vi "Conditioning.vi"() -> ()   [LabVIEW 2014]
uses:
  Licker.lvclass
  Juicer.lvclass
  Acquisition.lvclass
  Stimulus.lvclass
panel:
  out "Number of Licks":dbl[](array[numeric]) caption="#Licks"
  in  "LICK":bool[](array[boolean])=[FALSE, FALSE, FALSE, FALSE, FALSE]
  out "Last lick":timestamp[](array[timestamp])
  in  "IRI":dbl[](array[numeric]) caption="IRI (msec)"
  out "Time to stimulation":dbl[](array[numeric]) caption="Time to Stim"
  out "Rewards Given":dbl[](array[numeric]) caption="#Rew"
  in  "microL_per_pulse":dbl[](array[numeric]) caption="ml/p"
  in  "Pulse Duration":dbl[](array[numeric]) caption="Pulse (ms)"
  in  "Thr":dbl[](array[numeric])=[10.0, 10.0, 10.0, 10.0, 10.0]
  out "Water":bool[](array[boolean])
  out "Licks":bool[](array[boolean])
  out "error out":errorcluster
  in  "ITI":dbl[](array[numeric]) caption="ITI (min)"
  out "Stimulus":i32
  in  "RUN":bool[](array[boolean])=[FALSE, FALSE, FALSE, FALSE, FALSE]
  out "Licker":i32
  out "Acquisition":i32
  out "Juicer":i32
  in  "REC":bool[](array[boolean])=[FALSE, FALSE, FALSE, FALSE, FALSE]
  in  "liquid_type":string(combo)="water"
  in  "Type":enum16{"Calibrate", "Freerun", "BW"}[](array[ring])
  out "Optical traces":waveform(dbl)[](graph)
  in  "Mice ID":dbl[](array[numeric])
  in  "Stop":bool
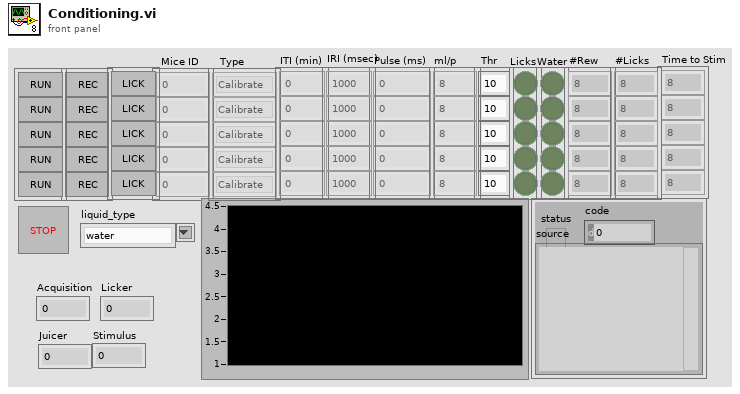
[diagram p1: front panel]
types:
  T1 = enum16{"stim_periods", "licks", "liquid_delivery"}
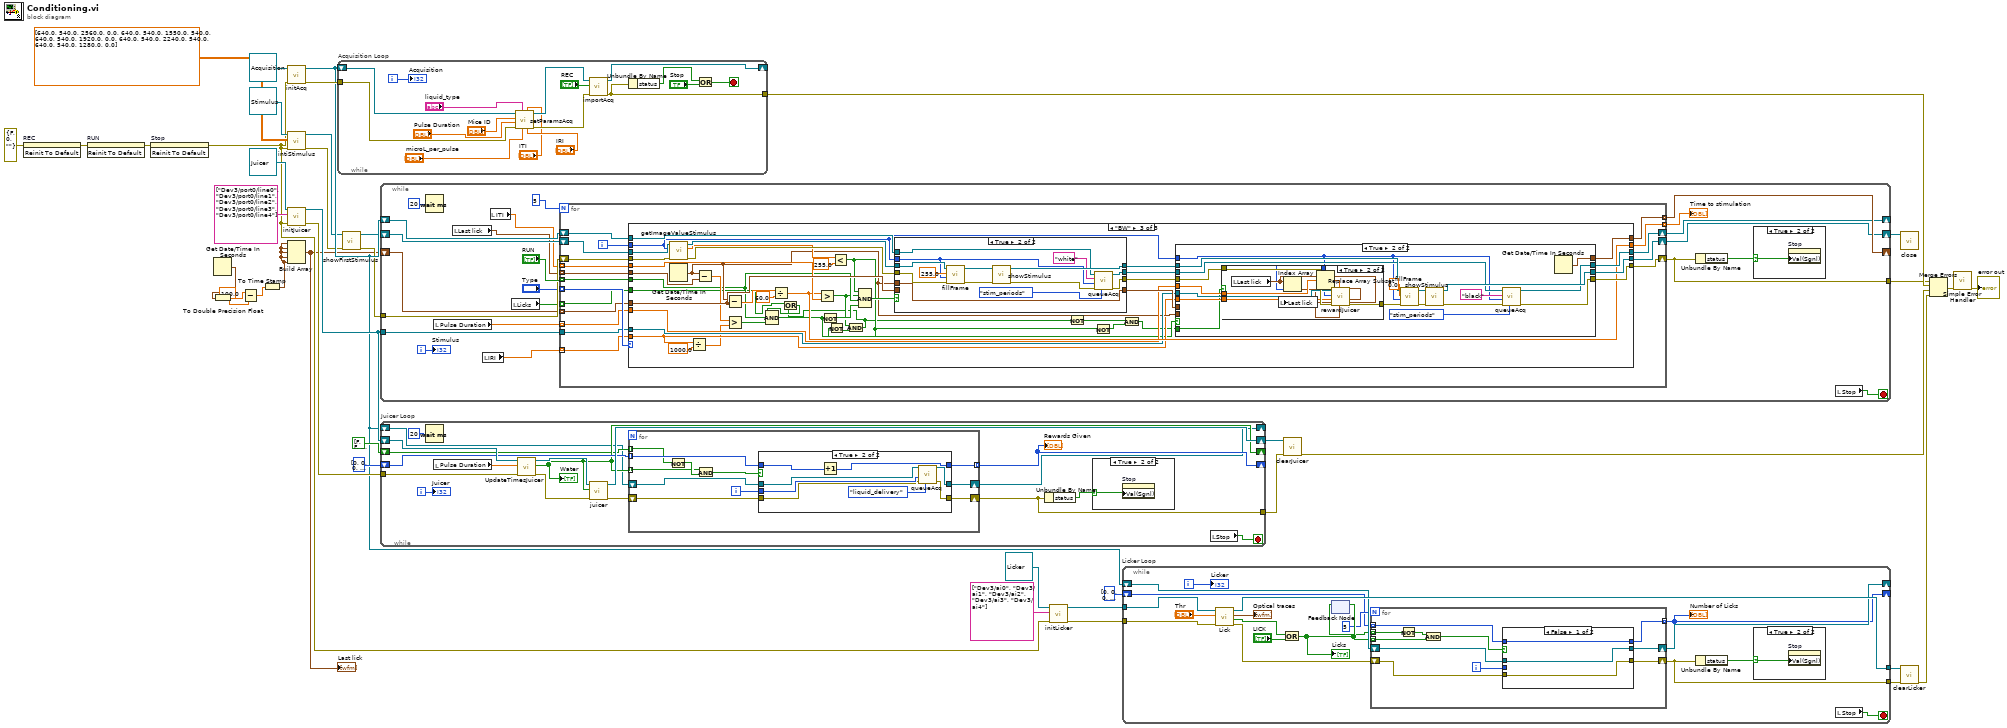
[diagram p0: block diagram]
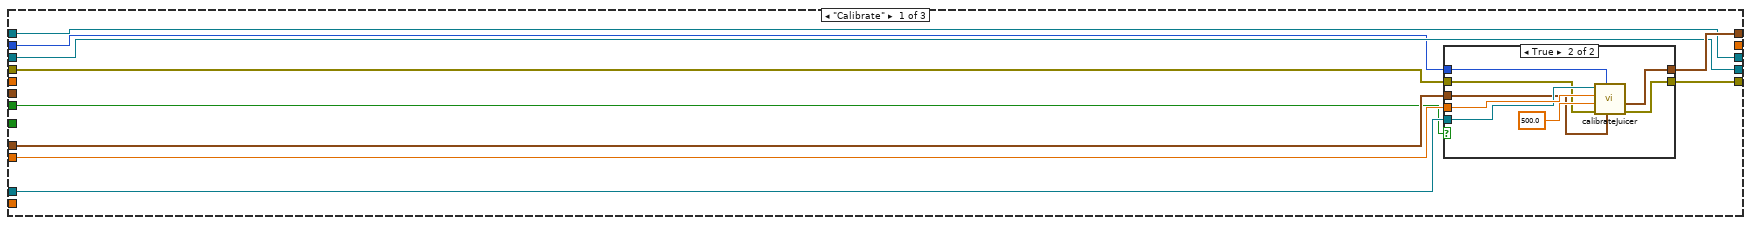
[diagram p3: hidden frame]
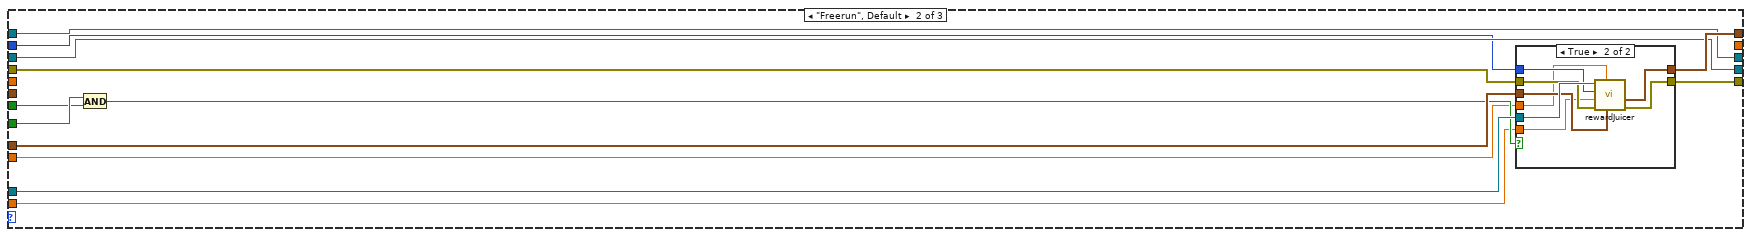
[diagram p5: hidden frame]
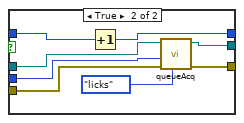
[diagram p11: hidden frame]
diagram:
  n1 = invoke on="REC" class="Arr (strict)" method="Reinit To Default"(error in=errorcluster {"status"=FALSE, "code"=0, "source"=""} ("error in (no error)")) -> (error out=w15:errorcluster)  [unwired: 2 in, 2 out]
  n2 = invoke on="RUN" class="Arr (strict)" method="Reinit To Default"(error in=w15) -> (error out=w14:errorcluster)  [unwired: 2 in, 2 out]
  n3 = invoke on="Stop" class="Bool (strict)" method="Reinit To Default"(error in=w14) -> (error out=w12:errorcluster)  [unwired: 2 in, 2 out]
  n4 = Get Date/Time In Seconds() -> (seconds since 1Jan1904=w4:timestamp)
  n5 = To Double Precision Float(number=w4) -> (double precision float=w3:dbl)
  n6 = Subtract(x=w3, y=100.0) -> (x-y=w1:dbl)
  n7 = To Time Stamp(1:w1) -> (0:w5:timestamp)
  n8 = call-dynamic "initAcq.vi"("error in (no error)"=w12, "Acquisition in"=refnum<class "Acquisition.lvclass"> refnum ("Acquisition.lvclass")) -> ("error out"=w32:errorcluster, "Acquisition out"=w16:refnum<class "Acquisition.lvclass">)  [unwired: 8 in]
  n9 = call-dynamic "intiStimulus.vi"("error in (no error)"=w12, "Monitor parameters"=dbl[][] [[640.0, 540.0, 2560.0, 0.0], [640.0, 540.0, 1550.0, 540.0], [640.0, 540.0, 1920.0, 0.0], [640.0, 540.0, 2240.0, 540.0], [640.0, 540.0, 1280.0, 0.0]], "Stimulus in"=refnum<class "Stimulus.lvclass"> refnum ("Stimulus.lvclass")) -> ("error out"=w10:errorcluster, "Stimulus out"=w11:refnum<class "Stimulus.lvclass">)  [unwired: 7 in]
  n10 = call-dynamic "initJuicer.vi"("error in (no error)"=w12, "Lines"=string[] ["Dev3/port0/line0", "Dev3/port0/line1", "Dev3/port0/line2", "Dev3/port0/line3", "Dev3/port0/line4"], "Juicer in"=refnum<class "Juicer.lvclass"> refnum ("Juicer.lvclass")) -> ("error out"=w36:errorcluster, "Juicer out"=w22:refnum<class "Juicer.lvclass">)  [unwired: 7 in]
  n11 = Build Array(w5, w5, w5, w5, w5) -> (w7:timestamp[])
  "Last lick" <- w7
  n12 = while "Acquisition Loop" {
    tunnel: w32 -> [w51]
    tunnel: [w45] -> w28
    shift-right: [w46] -> _
    shift-left: w16 -> [w58]
    i -> [w47]
    stop <- w49 stop-if-true
    n13 = call-dynamic "setParamsAcq.vi"("IRI"="IRI", "ITI"="ITI", "microL_per_pulse"="microL_per_pulse", "liquid_type"="liquid_type", "error in (no error)"=w51, "Pulse Duration"="Pulse Duration", "Mice ID"="Mice ID", "Acquisition in"=w58) -> ("error out"=w52:errorcluster, "Acquisition out"=w57:refnum<class "Acquisition.lvclass">)  [unwired: 2 in]
    n14 = call-dynamic "importAcq.vi"("error in (no error)"=w52, "REC"="REC", "Acquisition in"=w57) -> ("error out"=w45:errorcluster, "Acquisition out"=w46:refnum<class "Acquisition.lvclass">)  [unwired: 7 in]
    n15 = Unbundle By Name(w45) -> ("status"=w44:bool)
    n16 = Or(x=w44, y="Stop") -> (x .or. y?=w49:bool)
    "Acquisition" <- w47
  }
  n17 = call-dynamic "showFirstStimulus.vi"("error in (no error)"=w10, "Stimulus in"=w11) -> ("error out"=w9:errorcluster, "Stimulus out"=w8:refnum<class "Stimulus.lvclass">)  [unwired: 8 in]
  n18 = while {
    tunnel: w22 -> [w79]
    tunnel: w9 -> [w78]
    shift-right: [w74] -> _
    shift-left: w7 -> [w75]
    tunnel: [w62] -> w18
    shift-right: [w66] -> _
    shift-left: w16 -> [w67]
    shift-right: [w71] -> w19
    shift-left: w8 -> [w72]
    i -> [w69]
    stop <- w70 stop-if-true
    n19 = Wait (ms)(milliseconds to wait=u32 20) -> ()  [unwired: 1 out]
    n20 = local read "Pulse Duration"() -> (w77:dbl[])
    n21 = local read "Last lick"() -> (w64:timestamp[])
    n22 = local read "IRI"() -> (w60:dbl[])
    n23 = local read "ITI"() -> (w59:dbl[])
    n24 = local read "Licks"() -> (w76:bool[])
    n25 = for {
      N: 5 -> [_]
      tunnel: "RUN" -> [w92] mode=indexing
      tunnel: "Type" -> [w99] mode=indexing
      tunnel: w79 -> [w98]
      tunnel: w77 -> [w96] mode=indexing
      tunnel: w76 -> [w95] mode=indexing
      tunnel: w75 -> [w94] mode=indexing
      tunnel: [w93] -> w74 mode=indexing
      shift-right: [w89] -> w62
      shift-left: w78 -> [w97]
      tunnel: w59 -> [w87] mode=indexing
      shift-right: [w86] -> w66
      shift-left: w67 -> [w85]
      shift-right: [w90] -> w71
      shift-left: w72 -> [w91]
      tunnel: [w84] -> w65 mode=indexing
      tunnel: w60 -> [w83] mode=indexing
      tunnel: w64 -> [w82] mode=indexing
      i -> [w88]
      n26 = case shown="\"BW\"" w99 {
        tunnel: [w106 w130 w181] -> w89
        tunnel: w97 -> [w107 w131 w167]
        tunnel: w98 -> [w108 w132 w171]
        tunnel: w96 -> [w109 w120 w170]
        tunnel: w95 -> [_ w126 w151]
        tunnel: w94 -> [w105 w129 w182]
        tunnel: [w104 w128 w180] -> w93
        tunnel: w92 -> [w103 w125 w157]
        tunnel: w91 -> [w102 w124 w169]
        tunnel: [w102 w124 w179] -> w90
        tunnel: w88 -> [w100 w123 w162]
        tunnel: w85 -> [w101 w122 w178]
        tunnel: w87 -> [_ _ w176]
        tunnel: [w101 w122 w175] -> w86
        tunnel: [_ _ w172] -> w84
        tunnel: w83 -> [_ w121 w154]
        tunnel: w82 -> [_ _ w159]
        frame "Calibrate" {
          n27 = case shown="True" w103 {
            tunnel: w109 -> [_ w119]
            tunnel: w108 -> [_ w117]
            tunnel: w107 -> [w110 w116]
            tunnel: [w110 w115] -> w106
            tunnel: w105 -> [w111 w114]
            tunnel: [w111 w113] -> w104
            tunnel: w100 -> [_ w112]
            frame False {
            }
            frame True {
              n28 = call-dynamic "calibrateJuicer.vi"("Time Stamp"=w114, "Window Number (0...15)"=w112, "error in (no error)"=w116, "ISI"=500.0, "Pulse duration"=w119, "Juicer in"=w117) -> ("error out"=w115:errorcluster, "Time Stamp 2"=w113:timestamp)  [unwired: 3 in, 1 out]
            }
          }
        }
        frame "Freerun", Default {
          n29 = And(x=w126, y=w125) -> (x .and. y?=w127:bool)
          n30 = case shown="True" w127 {
            tunnel: w132 -> [_ w142]
            tunnel: w123 -> [_ w141]
            tunnel: w131 -> [w134 w140]
            tunnel: [w134 w139] -> w130
            tunnel: w129 -> [w133 w138]
            tunnel: [w133 w137] -> w128
            tunnel: w121 -> [_ w136]
            tunnel: w120 -> [_ w135]
            frame False {
            }
            frame True {
              n31 = call-dynamic "rewardJuicer.vi"("seconds since 1Jan1904 2"=w138, "pulse dur"=w135, "error in (no error)"=w140, "IRI"=w136, "Window Number (0...15)"=w141, "Juicer in"=w142) -> ("error out"=w139:errorcluster, "seconds since 1Jan1904"=w137:timestamp)  [unwired: 3 in, 1 out]
            }
          }
        }
        frame "BW" {
          n32 = call-dynamic "getImageValueStimulus.vi"("error in (no error)"=w167, "index"=w162, "Stimulus in"=w169) -> ("error out"=w166:errorcluster, "Pixel Value (Float)"=w164:sgl, "Stimulus out"=w168:refnum<class "Stimulus.lvclass">)  [unwired: 6 in]
          n33 = Get Date/Time In Seconds() -> (seconds since 1Jan1904=w161:timestamp)
          n34 = Divide(x=w154, y=1000.0) -> (x/y=w153:dbl)
          n35 = Subtract(x=w161, y=w159) -> (x-y=w160:dbl)
          n36 = Subtract(x=w161, y=w182) -> (x-y=w174:dbl)
          n37 = Greater?(x=w160, y=w153) -> (0:w158:bool)
          n38 = Divide(x=w174, y=60.0) -> (x/y=w172:dbl)
          n39 = Greater?(x=w172, y=w176) -> (0:w149:bool)
          n40 = Less?(x=w164, y=sgl 255.0) -> (x < y?=w147:bool)
          n41 = Not(x=w147) -> (.not. x?=w148:bool)
          n42 = And(x=w149, y=w148) -> (x .and. y?=w144:bool)
          n43 = Or(x=w151, y=w144) -> (x .or. y?=w150:bool)
          n44 = Compound Arithmetic op=AND(w150, w157, w158) -> (w152:bool)
          n45 = Not(x=w152) -> (.not. x?=w156:bool)
          n46 = Compound Arithmetic op=AND(w147, w149, w157, w156) -> (w165:bool)
          n47 = case shown="True" w165 {
            tunnel: [w221 w237] -> w185
            tunnel: [w222 w228] -> w184
            tunnel: w182 -> [w223 _]
            tunnel: [w223 w233] -> w183
            tunnel: w161 -> [_ w233]
            tunnel: w166 -> [w222 w232]
            tunnel: w168 -> [w221 w231]
            tunnel: w162 -> [_ w230]
            tunnel: w178 -> [w220 w227]
            tunnel: [w220 w226] -> w177
            frame False {
            }
            frame True {
              n48 = call-dynamic "fillFrame.vi"("error in (no error)"=w232, "index"=w230, "Pixel Value (U8, U16, I16, Float)"=sgl 255.0, "Stimulus in"=w231) -> ("error out"=w234:errorcluster, "Stimulus out"=w236:refnum<class "Stimulus.lvclass">)  [unwired: 6 in]
              n49 = call-dynamic "showStimulus.vi"("error in (no error)"=w234, "Stimulus in"=w236) -> ("error out"=w229:errorcluster, "Stimulus out"=w237:refnum<class "Stimulus.lvclass">)  [unwired: 8 in]
              n50 = call-dynamic "queueAcq.vi"("table"=T1."stim_periods", "error in (no error)"=w229, "Window Number (0...15)"=w230, "period_type"="white", "Acquisition in"=w227) -> ("error out"=w228:errorcluster, "Acquisition out"=w226:refnum<class "Acquisition.lvclass">)  [unwired: 4 in, 1 out]
            }
          }
          n51 = Not(x=w144) -> (.not. x?=w143:bool)
          n52 = Not(x=w147) -> (.not. x?=w146:bool)
          n53 = And(x=w143, y=w146) -> (x .and. y?=w145:bool)
          n54 = case shown="True" w152 {
            tunnel: w185 -> [w189 w205]
            tunnel: [w189 w204] -> w179
            tunnel: w184 -> [w188 w196]
            tunnel: [w188 w201] -> w181
            tunnel: [w187 w203] -> w180
            tunnel: w183 -> [w187 _]
            tunnel: w177 -> [w186 w200]
            tunnel: w162 -> [_ w191]
            tunnel: [w186 w197] -> w175
            tunnel: w171 -> [_ w194]
            tunnel: w161 -> [_ _]
            tunnel: w170 -> [_ w193]
            tunnel: w154 -> [_ w192]
            tunnel: w145 -> [_ w190]
            frame False {
            }
            frame True {
              n55 = case shown="True" w190 {
                tunnel: w196 -> [w209 w219]
                tunnel: [w209 w218] -> w195
                tunnel: w194 -> [_ w217]
                tunnel: w193 -> [_ w216]
                tunnel: w192 -> [_ w215]
                tunnel: w191 -> [_ w211]
                frame False {
                }
                frame True {
                  n56 = local read "Last lick"() -> (w212:timestamp[])
                  n57 = Index Array(array=w212, index=w211) -> (element=w210:timestamp)
                  n58 = call-dynamic "rewardJuicer.vi"("seconds since 1Jan1904 2"=w210, "pulse dur"=w216, "error in (no error)"=w219, "IRI"=w215, "Window Number (0...15)"=w211, "Juicer in"=w217) -> ("error out"=w218:errorcluster, "seconds since 1Jan1904"=w213:timestamp)  [unwired: 3 in, 1 out]
                  n59 = Replace Array Subset(array=w212, new element=w213, index=w211) -> (w214:timestamp[])
                  n60 = local write "Last lick"(w214) -> ()
                }
              }
              n61 = call-dynamic "fillFrame.vi"("error in (no error)"=w195, "index"=w191, "Pixel Value (U8, U16, I16, Float)"=sgl 0.0, "Stimulus in"=w205) -> ("error out"=w206:errorcluster, "Stimulus out"=w208:refnum<class "Stimulus.lvclass">)  [unwired: 6 in]
              n62 = call-dynamic "showStimulus.vi"("error in (no error)"=w206, "Stimulus in"=w208) -> ("error out"=w202:errorcluster, "Stimulus out"=w204:refnum<class "Stimulus.lvclass">)  [unwired: 8 in]
              n63 = call-dynamic "queueAcq.vi"("table"=T1."stim_periods", "error in (no error)"=w202, "Window Number (0...15)"=w191, "period_type"="black", "Acquisition in"=w200) -> ("error out"=w201:errorcluster, "Acquisition out"=w197:refnum<class "Acquisition.lvclass">)  [unwired: 4 in, 1 out]
              n64 = Get Date/Time In Seconds() -> (seconds since 1Jan1904=w203:timestamp)
            }
          }
        }
      }
    }
    "Time to stimulation" <- w65
    n65 = Unbundle By Name(w62) -> ("status"=w61:bool)
    n66 = case shown="True" w61 {
      selector: w61 -> [_ w81]
      frame False {
      }
      frame True {
        n67 = property on="Stop" class="Bool (strict)"("Val(Sgnl)"=w81) -> ()  [unwired: 2 in, 2 out]
      }
    }
    n68 = local read "Stop"() -> (w70:bool)
    "Stimulus" <- w69
  }
  n69 = while "Juicer Loop" {
    tunnel: [w245] -> w37
    tunnel: w36 -> [w250]
    shift-right: [w252] -> w38
    shift-left: w22 -> [w253]
    shift-right: [w242] -> _
    shift-left: i32[] [0, 0, 0, 0, 0] ("Array") -> [w243]
    shift-right: [w241] -> _
    shift-left: bool[] [FALSE, FALSE, FALSE, FALSE, FALSE] ("Juice") -> [w240]
    shift-right: [w238] -> _
    shift-left: w16 -> [w239]
    i -> [w246]
    stop <- w255 stop-if-true
    n70 = Wait (ms)(milliseconds to wait=u32 20) -> ()  [unwired: 1 out]
    n71 = local read "Pulse Duration"() -> (w247:dbl[])
    n72 = call-dynamic "UpdateTimesJuicer.vi"("error in (no error)"=w250, "Pulse Duration"=w247, "Juicer in"=w253) -> ("error out"=w251:errorcluster, "Juice"=w241:bool[], "Juicer out"=w254:refnum<class "Juicer.lvclass">)  [unwired: 6 in]
    "Water" <- w241
    n73 = call-dynamic "juicer.vi"("error in (no error)"=w251, "data"=w241, "Juicer in"=w254) -> ("error out"=w249:errorcluster, "Juicer out"=w252:refnum<class "Juicer.lvclass">)  [unwired: 7 in]
    n74 = for {
      tunnel: w241 -> [w265] mode=indexing
      shift-right: [w263] -> w245
      shift-left: w249 -> [w264]
      tunnel: w243 -> [w262] mode=indexing
      tunnel: [w261] -> w242 mode=indexing
      tunnel: w240 -> [w260] mode=indexing
      shift-right: [w258] -> w238
      shift-left: w239 -> [w259]
      i -> [w257]
      n75 = Not(x=w260) -> (.not. x?=w266:bool)
      n76 = And(x=w265, y=w266) -> (x .and. y?=w267:bool)
      n77 = case shown="True" w267 {
        tunnel: w257 -> [_ w277]
        tunnel: w264 -> [w270 w276]
        tunnel: [w270 w275] -> w263
        tunnel: w262 -> [w269 w274]
        tunnel: [w269 w273] -> w261
        tunnel: w259 -> [w268 w272]
        tunnel: [w268 w271] -> w258
        frame False {
        }
        frame True {
          n78 = Increment(x=w274) -> (x+1=w273:i32)
          n79 = call-dynamic "queueAcq.vi"("table"=T1."liquid_delivery", "error in (no error)"=w276, "Window Number (0...15)"=w277, "Acquisition in"=w272) -> ("error out"=w275:errorcluster, "Acquisition out"=w271:refnum<class "Acquisition.lvclass">)  [unwired: 5 in, 1 out]
        }
      }
    }
    "Rewards Given" <- w242
    n80 = Unbundle By Name(w245) -> ("status"=w244:bool)
    n81 = case shown="True" w244 {
      selector: w244 -> [_ w256]
      frame False {
      }
      frame True {
        n82 = property on="Stop" class="Bool (strict)"("Val(Sgnl)"=w256) -> ()  [unwired: 2 in, 2 out]
      }
    }
    n83 = local read "Stop"() -> (w255:bool)
    "Juicer" <- w246
  }
  n84 = call-dynamic "initLicker.vi"("error in (no error)"=w12, "Lines"=string[] ["Dev3/ai0", "Dev3/ai1", "Dev3/ai2", "Dev3/ai3", "Dev3/ai4"], "Licker in"=refnum<class "Licker.lvclass"> refnum ("Licker.lvclass")) -> ("error out"=w34:errorcluster, "Licker out"=w39:refnum<class "Licker.lvclass">)  [unwired: 7 in]
  n85 = while "Licker Loop" {
    tunnel: w34 -> [w294]
    tunnel: [w279] -> w31
    tunnel: w39 -> [w296]
    tunnel: [w295] -> w35
    shift-right: [w286] -> _
    shift-left: w16 -> [w287]
    shift-right: [w280] -> _
    shift-left: i32[] [0, 0, 0, 0, 0] ("Array") -> [w281]
    i -> [w290]
    stop <- w297 stop-if-true
    n86 = call-dynamic "Lick.vi"("error in (no error)"=w294, "% decrease Thr"="Thr", "Licker in"=w296) -> ("error out"=w291:errorcluster, "Lick?"=w288:bool[], "data"=→"Optical traces":waveform(dbl)[], "Licker out"=w295:refnum<class "Licker.lvclass">)  [unwired: 5 in]
    n87 = Or(x=w288, y="LICK") -> (x .or. y?=w285:bool[])
    "Licks" <- w285
    n88 = feedback-in #1(w285) -> ()
    n89 = feedback #1() -> (w284:bool[])  [unwired: 1 in]
    n90 = for {
      N: 5 -> [_]
      tunnel: w285 -> [w304] mode=indexing
      shift-right: [w308] -> w279
      shift-left: w291 -> [w309]
      shift-right: [w306] -> w286
      shift-left: w287 -> [w307]
      tunnel: w284 -> [w303] mode=indexing
      tunnel: w281 -> [w300] mode=indexing
      tunnel: [w299] -> w280 mode=indexing
      i -> [w305]
      n91 = Not(x=w303) -> (.not. x?=w302:bool)
      n92 = And(x=w302, y=w304) -> (x .and. y?=w301:bool)
      n93 = case shown="False" w301 {
        tunnel: w305 -> [_ w315]
        tunnel: w309 -> [w312 w319]
        tunnel: [w312 w318] -> w308
        tunnel: w307 -> [w311 w317]
        tunnel: [w311 w316] -> w306
        tunnel: w300 -> [w310 w314]
        tunnel: [w310 w313] -> w299
        frame False {
        }
        frame True {
          n94 = Increment(x=w314) -> (x+1=w313:i32)
          n95 = call-dynamic "queueAcq.vi"("table"=T1."licks", "error in (no error)"=w319, "Window Number (0...15)"=w315, "Acquisition in"=w317) -> ("error out"=w318:errorcluster, "Acquisition out"=w316:refnum<class "Acquisition.lvclass">)  [unwired: 5 in, 1 out]
        }
      }
    }
    "Number of Licks" <- w280
    n96 = Unbundle By Name(w279) -> ("status"=w289:bool)
    n97 = case shown="True" w289 {
      selector: w289 -> [_ w298]
      frame False {
      }
      frame True {
        n98 = property on="Stop" class="Bool (strict)"("Val(Sgnl)"=w298) -> ()  [unwired: 2 in, 2 out]
      }
    }
    n99 = local read "Stop"() -> (w297:bool)
    "Licker" <- w290
  }
  n100 = call-dynamic "clearJuicer.vi"("error in (no error)"=w37, "Juicer in"=w38) -> ("error out"=w29:errorcluster)  [unwired: 8 in, 1 out]
  n101 = call-dynamic "close.vi"("Stimulus in"=w19) -> ()  [unwired: 9 in, 2 out]
  n102 = call-dynamic "clearLicker.vi"("error in (no error)"=w31, "Licker in"=w35) -> ("error out"=w30:errorcluster)  [unwired: 8 in, 1 out]
  n103 = Merge Errors(w18, w28, w29, w30) -> (w27:errorcluster)
  n104 = call <vilib>:"Simple Error Handler.vi"("error in (no error)"=w27) -> ("error out"=→"error out":errorcluster)  [unwired: 4 in, 4 out]
